vi "calc2019.vi"() -> ()   [LabVIEW 2017]
uses:
  <vilib>/gmath/NI_Gmath.lvlib
panel:
  out "Boolean Text.Text":string
  out "String":string
  in  "button =":bool
  in  "button -":bool
  in  "button +":bool
  in  "button 9":bool
  in  "button 8":bool
  in  "button 7":bool
  in  "button 6":bool
  in  "button 5":bool
  in  "button 4":bool
  in  "button 3":bool
  in  "button 2":bool
  in  "button 1":bool
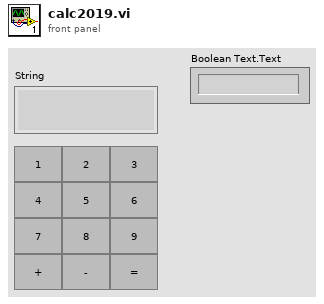
[diagram p1: front panel]
types:
  T1 = typedef "eventvkey.ctl" = enum16{"ASCII", "Enter", "Return", "Shift", "Ctrl", "Alt", "Cmd", "Opt", "Caps", "NumLock", "Clear", "Break", "Up", "Down", "Left", "Right", "Insert", "Delete", "Home", "End", "PageUp", "PageDown", "Escape", "Help", "Pause", "ScrollLock", "F1", "F2", "F3", "F4", "F5", "F6", "F7", "F8", "F9", "F10", "F11", "F12", "F13", "F14", "F15", "F16", "F17", "F18", "F19", "F20", "F21", "F22", "F23", "F24", "Play", "VolumeUp", "VolumeDown", "Mute", "Two Byte Char"}
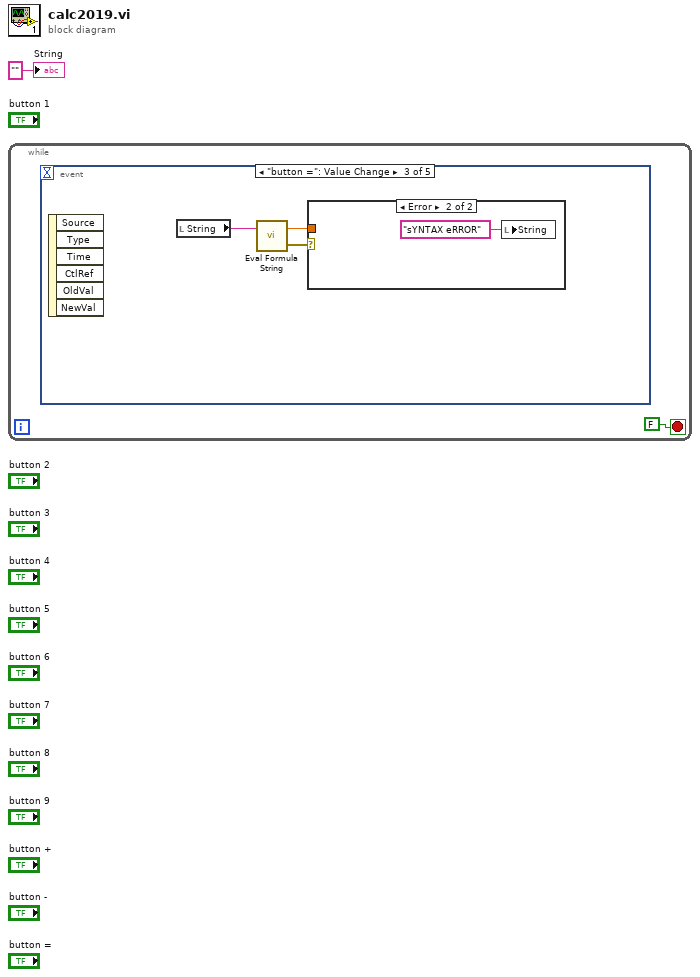
[diagram p0: block diagram]
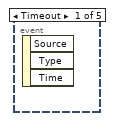
[diagram p2: hidden frame]
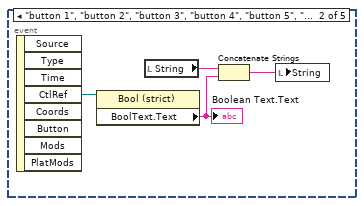
[diagram p3: hidden frame]
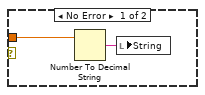
[diagram p4: hidden frame]
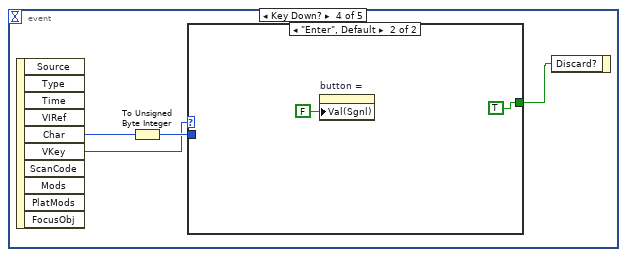
[diagram p5: hidden frame]
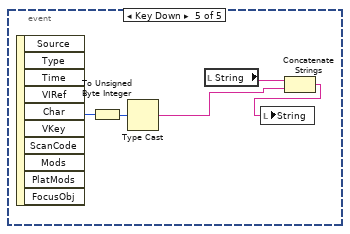
[diagram p7: hidden frame]
diagram:
  n1 = while {
    stop <- FALSE stop-if-true
    n2 = event shown="[2] \"button =\": Value Change" {
      selector: _ -> [_ _ _ _ _]
      dyn-events: _ -> [_ _ _ _ _]
      timeout: _ -> [_ _ _ _ _]
      event Timeout {
        n3 = event-data() -> ()  [unwired: 1 in, 3 out]
      }
      event "button 1", "button 2", "button 3", "button 4", "button 5", "button 6", "button 7", "button 8", "button 9", "button +", "button -": Mouse Down {
        n4 = event-data() -> ("CtlRef"=w6:refnum<vi>)  [unwired: 1 in, 7 out]
        n5 = property class="Bool (strict)"(reference=w6) -> ("BoolText.Text"=w4:string)  [unwired: 1 in, 2 out]
        "Boolean Text.Text" <- w4
        n6 = local read "String"() -> (w5:string)
        n7 = Concatenate Strings(w5, w4) -> (w3:string)
        n8 = local write "String"(w3) -> ()
      }
      event "button =": Value Change {
        n9 = event-data() -> ()  [unwired: 1 in, 6 out]
        n10 = local read "String"() -> (w9:string)
        n11 = call <vilib>:"Eval Formula String.vi"("formula"=w9) -> ("error out"=w8:errorcluster, "y value"=w7:dbl)  [unwired: 1 in]
        n12 = case shown="Error" w8 {
          tunnel: w7 -> [w11 _]
          frame No Error {
            n13 = Number To Decimal String(number=w11) -> (decimal integer string=w10:string)  [unwired: 1 in]
            n14 = local write "String"(w10) -> ()
          }
          frame Error {
            n15 = local write "String"("sYNTAX eRROR" ("String")) -> ()
          }
        }
      }
      event Key Down? {
        n16 = event-data() -> ("Char"=w16:i16, "VKey"=w13:T1)  [unwired: 1 in, 8 out]
        n17 = To Unsigned Byte Integer(number=w16) -> (unsigned 8bit integer=w15:u8)
        n18 = case shown="\"Enter\", Default" w13 {
          tunnel: w15 -> [_ _]
          tunnel: [_ TRUE] -> w14
          frame "ASCII", "Shift" {
          }
          frame "Enter", Default {
            n19 = property on="button =" class="Bool (strict)"("Val(Sgnl)"=FALSE ("Value (Signaling)")) -> ()  [unwired: 2 in, 2 out]
          }
        }
        n20 = event-data("Discard?"=w14) -> ()  [unwired: 1 in, 1 out]
      }
      event Key Down {
        n21 = event-data() -> ("Char"=w22:i16)  [unwired: 1 in, 9 out]
        n22 = To Unsigned Byte Integer(number=w22) -> (unsigned 8bit integer=w23:u8)
        n23 = Type Cast(x=w23) -> (*(type *) &x=w20:string)  [unwired: 1 in]
        n24 = local read "String"() -> (w21:string)
        n25 = Concatenate Strings(w21, w20) -> (w19:string)
        n26 = local write "String"(w19) -> ()
      }
    }
  }
  "String" <- "" ("String")
